vi "Create All Message Queues.vi"(8 "error in (no error)":errorcluster) -> (0 "error out":errorcluster, 3 "Message Queues out":T1)   [LabVIEW 2013, in "repositoryConfigurator Message Queue.lvlib"]
doc: "This VI creates and initializes all the message queues for your application. If your application requires more than one message queue, right-click the \"Message Queues\" constant above and select Open Type Def. Add the new Message Queue(s) to the type definition, then initialize them in this VI."
uses:
  repositoryConfigurator Message Queue.lvlib
  All Message Queues.ctl
  Message Cluster.ctl
  Enqueue Message (Single).vi
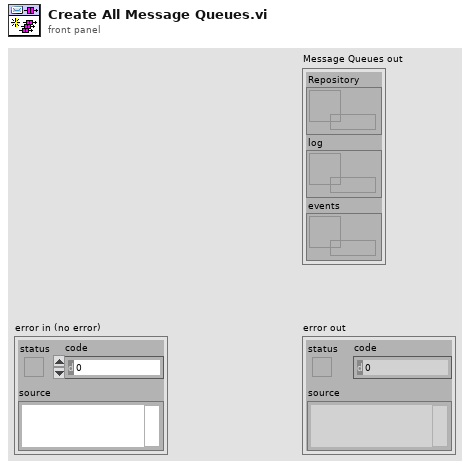
[diagram p1: front panel]
types:
  T1 = typedef "repositoryConfigurator Message Queue.lvlib/All Message Queues.ctl" = cluster{"Repository":refnum<queue>, "log":refnum<queue>, "events":refnum<queue>}
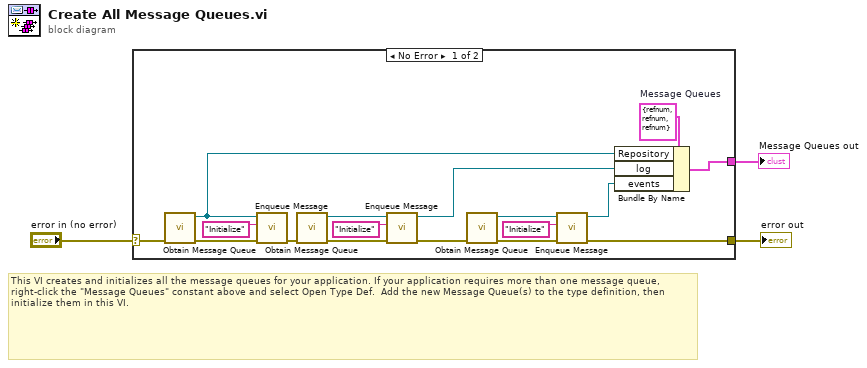
[diagram p0: block diagram]
diagram:
  # "This VI creates and initializes all the message queues for your application. If your application requires more than one message queue, right-click the \"Message Queues\" constant above and select Open Type Def.  Add the new Message Queue(s) to the type definition, then initialize them in this VI."
  n1 = case shown="No Error" "error in (no error)" {
    selector: "error in (no error)" -> [w18 w21]
    tunnel: [w5 w21] -> w3
    tunnel: [w19 _] -> w2
    frame No Error {
      w20 = T1 {"Repository"=refnum, "log"=refnum, "events"=refnum}  # Message Queues
      n2 = call "Obtain Message Queue.vi"("error in (no error)"=w18) -> ("error out"=w17:errorcluster, "Message Queue"=w15:refnum<queue>)  [unwired: 9 in]
      n3 = call-poly "Enqueue Message.vi"("error in (no error)"=w17, "Message"="Initialize", "Message Queue"=w15) -> ("error out"=w14:errorcluster)  [unwired: 7 in, 1 out]
      n4 = call "Obtain Message Queue.vi"("error in (no error)"=w14) -> ("error out"=w12:errorcluster, "Message Queue"=w10:refnum<queue>)  [unwired: 9 in]
      n5 = call-poly "Enqueue Message.vi"("error in (no error)"=w12, "Message"="Initialize", "Message Queue"=w10) -> ("error out"=w6:errorcluster, "dup Message Queue"=w11:refnum<queue>)  [unwired: 7 in]
      n6 = call "Obtain Message Queue.vi"("error in (no error)"=w6) -> ("error out"=w8:errorcluster, "Message Queue"=w9:refnum<queue>)  [unwired: 9 in]
      n7 = call-poly "Enqueue Message.vi"("error in (no error)"=w8, "Message"="Initialize", "Message Queue"=w9) -> ("error out"=w5:errorcluster, "dup Message Queue"=w4:refnum<queue>)  [unwired: 7 in]
      n8 = Bundle By Name(cluster=w20, "Repository"=w15, "log"=w11, "events"=w4) -> (w19:T1)
    }
    frame Error {
    }
  }
  "Message Queues out" <- w2
  "error out" <- w3
